vi "Test_Remain.vi"(3 "elapsed":i32, 4 "Period":u8, 5 "load":i32, 6 "preload":i32) -> (0 "used":string, 1 "Period":string, 2 "remain":string)   [LabVIEW 2015]
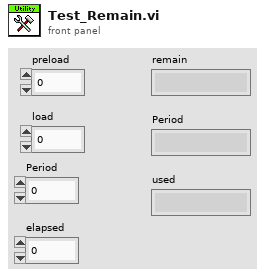
[diagram p1: front panel]
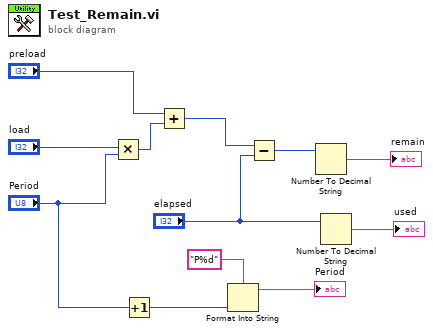
[diagram p0: block diagram]
diagram:
  n1 = Multiply(x="load", y="Period") -> (x*y=w10:i32)
  n2 = Increment(x="Period") -> (x+1=w1:u8)
  n3 = Add(x="preload", y=w10) -> (x+y=w7:i32)
  n4 = Format Into String(format string="P%d", w1) -> (resulting string=→"Period":string)  [unwired: 2 in, 1 out]
  n5 = Subtract(x=w7, y="elapsed") -> (x-y=w6:i32)
  n6 = Number To Decimal String(number=w6) -> (decimal integer string=→"remain":string)  [unwired: 1 in]
  n7 = Number To Decimal String(number="elapsed") -> (decimal integer string=→"used":string)  [unwired: 1 in]
